vi "ConnectedAxes.vi"() -> ()   [LabVIEW 2013]
panel:
  out "Connected Axes":string[](array[string])
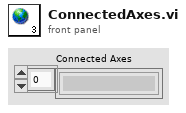
[diagram p1: front panel]
diagram:
